vi "Esercitazione 8 - Event Structure.vi"() -> ()   [LabVIEW 2018]
panel:
  out "NewVal":bool
  out "OldVal":bool
  in  "Stop Button":bool
  out "String":string
  in  "Mail Button":bool
  in  "Cancel Button":bool
  in  "Home Button":bool
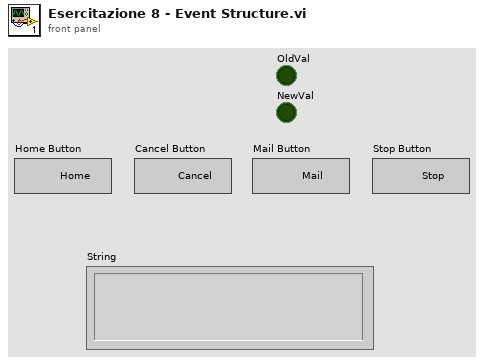
[diagram p1: front panel]
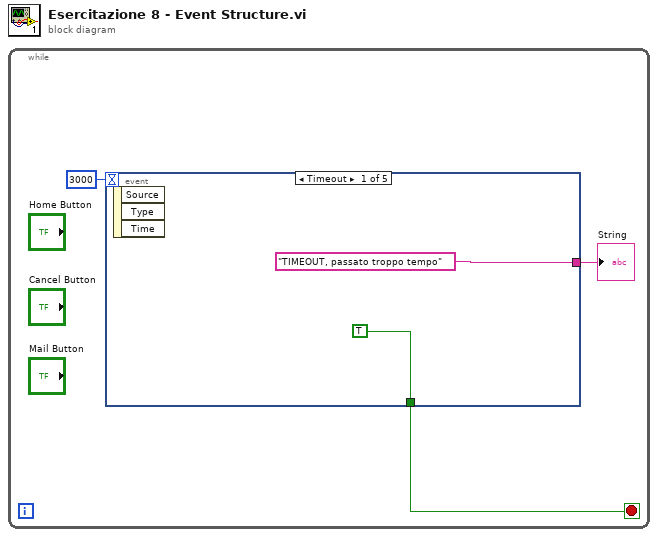
[diagram p0: block diagram]
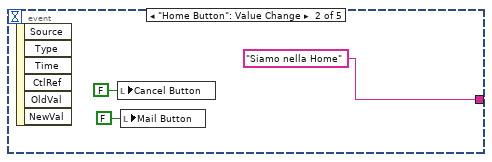
[diagram p2: hidden frame]
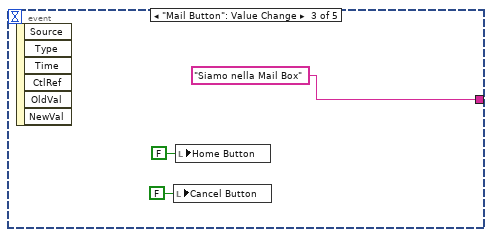
[diagram p3: hidden frame]
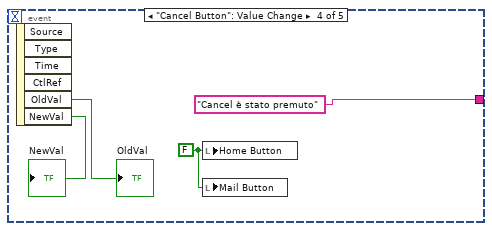
[diagram p4: hidden frame]
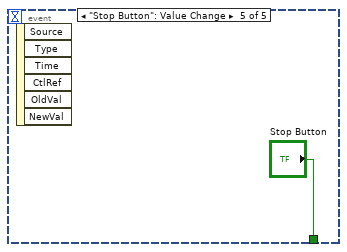
[diagram p5: hidden frame]
diagram:
  n1 = while {
    stop <- w2 stop-if-true
    n2 = event shown="[0] Timeout" {
      selector: _ -> [_ _ _ _ _]
      dyn-events: _ -> [_ _ _ _ _]
      timeout: 3000 -> [_ _ _ _ _]
      tunnel: ["TIMEOUT, passato troppo tempo" "Siamo nella Home" "Siamo nella Mail Box" "Cancel è stato premuto" _] -> w3
      tunnel: [TRUE _ _ _ "Stop Button"] -> w2
      event Timeout {
        n3 = event-data() -> ()  [unwired: 1 in, 3 out]
      }
      event "Home Button": Value Change {
        n4 = event-data() -> ()  [unwired: 1 in, 6 out]
        n5 = local write "Cancel Button"(FALSE ("Cancel Button")) -> ()
        n6 = local write "Mail Button"(FALSE ("Mail Button")) -> ()
      }
      event "Mail Button": Value Change {
        n7 = event-data() -> ()  [unwired: 1 in, 6 out]
        n8 = local write "Cancel Button"(FALSE ("Cancel Button")) -> ()
        n9 = local write "Home Button"(FALSE ("Home Button")) -> ()
      }
      event "Cancel Button": Value Change {
        w14 = FALSE ("Home Button")
        n10 = event-data() -> ("OldVal"=→"OldVal":bool, "NewVal"=→"NewVal":bool)  [unwired: 1 in, 4 out]
        n11 = local write "Home Button"(w14) -> ()
        n12 = local write "Mail Button"(w14) -> ()
      }
      event "Stop Button": Value Change {
        n13 = event-data() -> ()  [unwired: 1 in, 6 out]
      }
    }
    "String" <- w3
  }
